vi "Sense Hat Example.vi"() -> ()   [LabVIEW 2020]
uses:
  LINX-SenseHat/Barometer Readings.ctl
  LINX-SenseHat/HTS221 Data.ctl
  LINX-SenseHat/IMU Data.ctl
  LSM9DS1/3 Axis Values.ctl
  <vilib>/MakerHub/LINX/Public/Utilities/Open Local.vi
  <vilib>/MakerHub/LINX/LMH-LINX.lvlib
  LINX-SenseHat/LINX-SenseHat.lvclass
  LSM9DS1/LSM9DS1 IMU.lvclass
panel:
  out "IMU Data":T1
  out "Joystick Buttons":u8
  in  "LED Array":u32[][](array[colorbox])=[[0, 0, 0, 0, 0, 0, 0, 0], [0, 0, 0, 0, 0, 0, 0, 0], [0, 0, 0, 0, 0, 0, 0, 0], [0, 0, 0, 0, 0, 0, 0, 0], [0, 0, 0, 0, 0, 0, 0, 0], [0, 0, 0, 0, 0, 0, 0, 0], [0, 0, 0, 0, 0, 0, 0, 0], [0, 0, 0, 0, 0, 0, 0, 0]]
  out "HTS221 Data":T3
  out "LPS25H Data":T4
  out "Error Out":errorcluster
  in  "stop":bool
  # "Raspberry Pi Sense Hat Example"
  # "The Raspberry Pi Sense Hat includes:\n- LSM9DS1 9DOF IMU (Accelerometer, Gyroscope, Magnetometer)\n- LPS25H Barometer (Temperature & Pressure)\n- HTS221 Temperature/Humidity Sensor\n- Joystick with Push Button\n- 8x8 RGB LED Array"
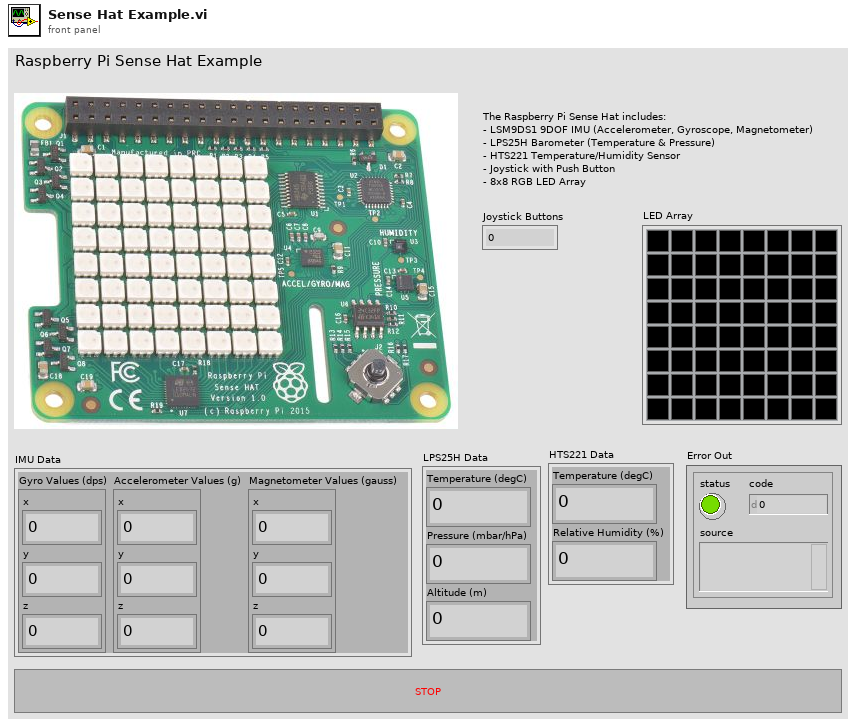
[diagram p1: front panel]
types:
  T1 = typedef "LINX-SenseHat.lvclass/IMU Data.ctl" = cluster{"Gyro Values (dps)":T2, "Accelerometer Values (g)":T2, "Magnetometer Values (gauss)":T2}
  T2 = typedef "LSM9DS1 IMU.lvclass/3 Axis Values.ctl" = cluster{"x":dbl, "y":dbl, "z":dbl}
  T3 = typedef "LINX-SenseHat.lvclass/HTS221 Data.ctl" = cluster{"Temperature (degC)":dbl, "Relative Humidity (%)":dbl}
  T4 = typedef "LINX-SenseHat.lvclass/Barometer Readings.ctl" = cluster{"Temperature (degC)":dbl, "Pressure (mbar/hPa)":dbl, "Altitude (m)":dbl}
  T5 = typedef "LMH-LINX.lvlib/LINX Ref.ctl" = cluster{"IO":T6, "Interface":T7, "LINX Device Config":T8}
  T6 = typedef "LMH-LINX.lvlib/Platform.ctl" = enum16{"Remote", "Local"}
  T7 = typedef "LMH-LINX.lvlib/Interface.ctl" = enum16{"Serial", "TCP"}
  T8 = typedef "LMH-LINX.lvlib/Device.lvlib/LINX Device Config.ctl" = cluster{"Interface":T7, "COM Port":refnum<visa-resource-name>, "TCP Configuration":T9, "Device Family":u8, "Device ID":u8, "Device Name":string, "TCP Ref":refnum<k5>, "Channels":T10}
  T9 = typedef "LMH-LINX.lvlib/Device.lvlib/TCP Config.ctl" = cluster{"IP Address":string, "Port":u16}
  T10 = typedef "LMH-LINX.lvlib/Channels.ctl" = cluster{"DI":u8[], "DO":u8[], "AI":u8[], "AO":u8[], "PWM":u8[], "QE":u8[], "UART":u8[], "I2C 2":u8[], "SPI":u8[], "CAN":u8[], "Servo":u8[], "AI Ref (V)":dbl, "AI Resolution (Bits)":u8, "AO Ref (V)":dbl, "AO Resolution (Bits)":u8}
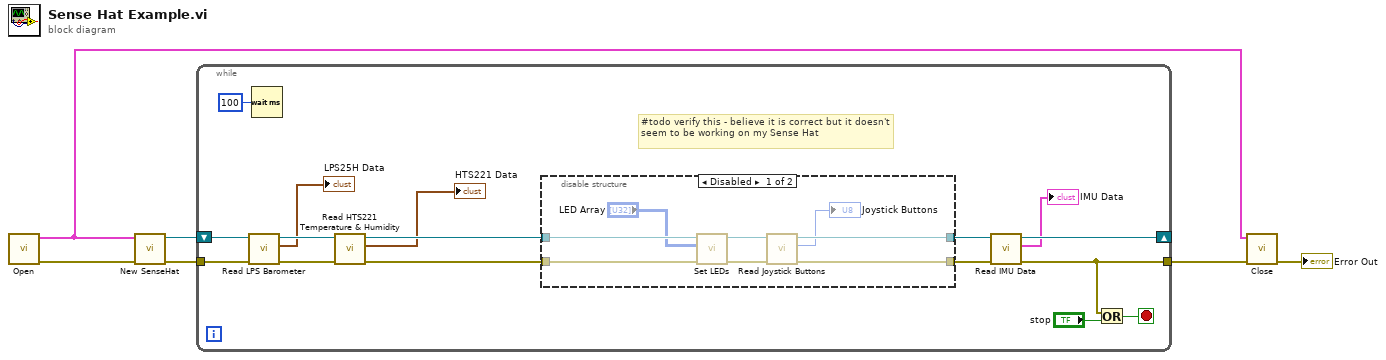
[diagram p0: block diagram]
diagram:
  n1 = call-poly <vilib>:"Open.vi"() -> ("Error Out"=w2:errorcluster, "LINX Resource"=w3:T5)  [unwired: 9 in, 1 out]
  n2 = call "New SenseHat.vi"("error in (no error)"=w2, "LINX Resource"=w3) -> ("error out"=w4:errorcluster, "LINX-SenseHat out"=w5:refnum<class "LINX-SenseHat.lvclass">)  [unwired: 8 in]
  n3 = while {
    tunnel: [w9] -> w1
    shift-right: [w8] -> _
    shift-left: w5 -> [w18]
    tunnel: w4 -> [w19]
    stop <- w21 stop-if-true
    # "#todo verify this - believe it is correct but it doesn't seem to be working on my Sense Hat"
    n4 = call "Read LPS Barometer.vi"("error in (no error)"=w19, "LINX-SenseHat in"=w18) -> ("error out"=w15:errorcluster, "LPS25H Readings"=→"LPS25H Data":T4, "LINX-SenseHat out"=w14:refnum<class "LINX-SenseHat.lvclass">)  [unwired: 7 in]
    n5 = Wait (ms)(milliseconds to wait=u32 100) -> ()  [unwired: 1 out]
    n6 = call "Read HTS221 Temperature & Humidity.vi"("error in (no error)"=w15, "LINX-SenseHat in"=w14) -> ("error out"=w17:errorcluster, "HTS221 Data"=→"HTS221 Data":T3, "LINX-SenseHat out"=w16:refnum<class "LINX-SenseHat.lvclass">)  [unwired: 7 in]
    n7 = disable-structure shown="Disabled" {
      disable-tunnel: w17 -> [w29 w31]
      disable-tunnel: w16 -> [w28 w32]
      disable-tunnel: [w27 w32] -> w11
      disable-tunnel: [w25 w31] -> w10
      frame Disabled {
        n8 = call "Set LEDs.vi"("error in (no error)"=w29, "LED Array"="LED Array", "LINX-SenseHat in"=w28) -> ("error out"=w26:errorcluster, "LINX-SenseHat out"=w30:refnum<class "LINX-SenseHat.lvclass">)  [unwired: 7 in]
        n9 = call "Read Joystick Buttons.vi"("error in (no error)"=w26, "LINX-SenseHat in"=w30) -> ("error out"=w25:errorcluster, "Joystick Buttons"=→"Joystick Buttons":u8, "LINX-SenseHat out"=w27:refnum<class "LINX-SenseHat.lvclass">)  [unwired: 7 in]
      }
      frame Enabled {
      }
    }
    n10 = call "Read IMU Data.vi"("error in (no error)"=w10, "LINX-SenseHat in"=w11) -> ("error out"=w9:errorcluster, "IMU Data"=→"IMU Data":T1, "LINX-SenseHat out"=w8:refnum<class "LINX-SenseHat.lvclass">)  [unwired: 7 in]
    n11 = Or(x=w9, y="stop") -> (x .or. y?=w21:bool)
  }
  n12 = call <vilib>:"Close.vi"("Error In"=w1, "LINX Resource"=w3) -> ("Error Out"=→"Error Out":errorcluster)  [unwired: 9 in]
